vi "setValue.vi"(8 "error in (no error)":errorcluster, 10 "Value":string="000000000000000000000000", 11 "tBSONObjectID in":refnum<class "tBSONObjectID.lvclass">) -> (0 "error out":errorcluster, 3 "tBSONObjectID out":refnum<class "tBSONObjectID.lvclass">)   [LabVIEW 2013, in "BSON.lvlib" / "tBSONObjectID.lvclass"]
uses:
  tBSONObjectID.lvclass
  status.ctl
  tBSONObjectID.lvclass/tBSONObjectID.ctl
  BSON.lvlib
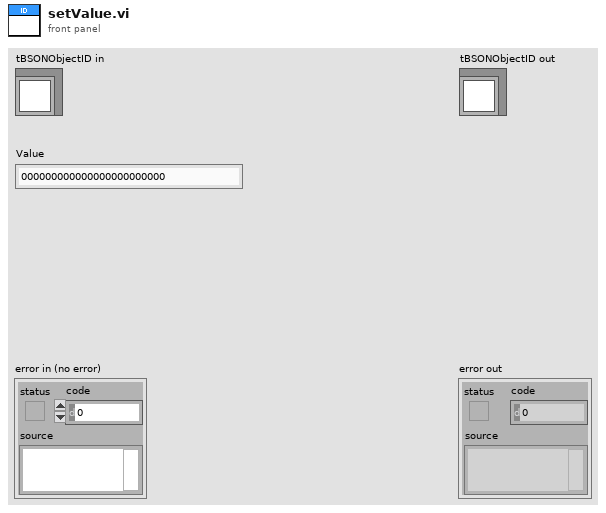
[diagram p1: front panel]
types:
  T1 = typedef "BSON.lvlib/status.ctl" = enum16{"Stream Corrupted or Ended Abruptly", "Incorrect Type In Stream", "ObjectID Invalid", "Method Not Implemented", "Invalid Name", "Invalid URI", "AutoReconnect", "Operation Failed", "Incorrectly Configured", "Cursor Not Found", "Timeout", "Invalid Type", "Empty Name", "Duplicate Name", "MD5Incorrect"}
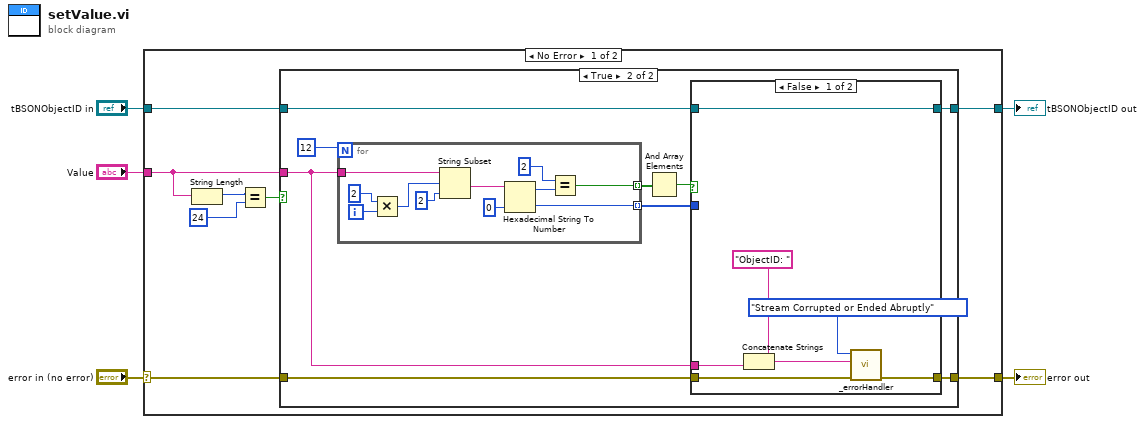
[diagram p0: block diagram]
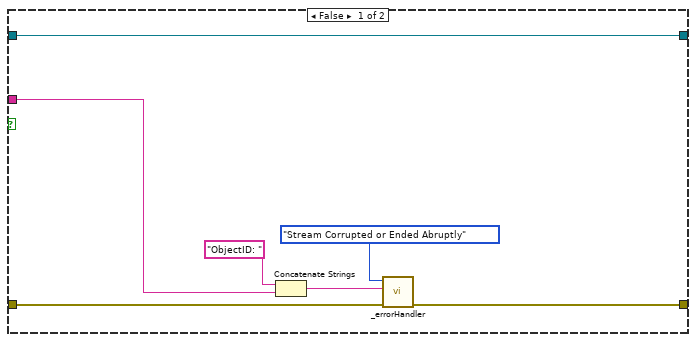
[diagram p2: hidden frame]
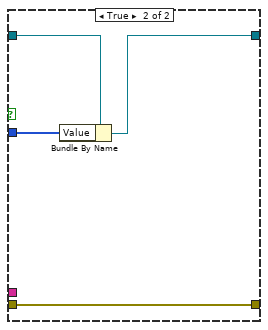
[diagram p3: hidden frame]
diagram:
  n1 = case shown="No Error" "error in (no error)" {
    selector: "error in (no error)" -> [w10 w53]
    tunnel: [w8 w53] -> w4
    tunnel: [w6 w52] -> w2
    tunnel: "tBSONObjectID in" -> [w7 w52]
    tunnel: "Value" -> [w11 _]
    frame No Error {
      n2 = String Length(string=w11) -> (length=w12:i32)
      n3 = Equal?(x=w12, y=24) -> (x = y?=w9:bool)
      n4 = case shown="True" w9 {
        tunnel: w11 -> [w14 w21]
        tunnel: w10 -> [w16 w23]
        tunnel: [w15 w22] -> w8
        tunnel: w7 -> [w20 w28]
        tunnel: [w20 w26] -> w6
        frame False {
          n5 = Concatenate Strings("ObjectID: " ("string"), w14) -> (w17:string)
          n6 = call "_errorHandler.vi"("error in (no error)"=w16, "Additional Text"=w17, "Error Type"=status."Stream Corrupted or Ended Abruptly") -> ("error out"=w15:errorcluster)  [unwired: 8 in]
        }
        frame True {
          n7 = for {
            N: 12 -> [_]
            tunnel: w21 -> [w51]
            tunnel: [w47] -> w27 mode=indexing
            tunnel: [w41] -> w25 mode=indexing
            i -> [w46]
            n8 = Multiply(x=2, y=w46) -> (x*y=w44:i32)
            n9 = String Subset(string=w51, offset (0)=w44, length (rest)=2 ("length (rest)")) -> (substring=w49:string)
            n10 = Hexadecimal String To Number(string=w49, default (0uL)=u8 0 ("default (0 U32)")) -> (offset past number=w43:i32, number=w47:u8)  [unwired: 1 in]
            n11 = Equal?(x=2, y=w43) -> (x = y?=w41:bool)
          }
          n12 = And Array Elements(Boolean array=w25) -> (logical AND=w24:bool)
          n13 = case shown="False" w24 {
            tunnel: w28 -> [w36 w40]
            tunnel: w27 -> [_ w39]
            tunnel: [w36 w38] -> w26
            tunnel: w23 -> [w35 w37]
            tunnel: [w34 w37] -> w22
            tunnel: w21 -> [w32 _]
            frame False {
              n14 = Concatenate Strings("ObjectID: " ("string"), w32) -> (w30:string)
              n15 = call "_errorHandler.vi"("error in (no error)"=w35, "Additional Text"=w30, "Error Type"=status."Stream Corrupted or Ended Abruptly") -> ("error out"=w34:errorcluster)  [unwired: 8 in]
            }
            frame True {
              n16 = Bundle By Name(cluster=w40, "Value"=w39) -> (w38:refnum<class "tBSONObjectID.lvclass">)
            }
          }
        }
      }
    }
    frame Error {
    }
  }
  "error out" <- w4
  "tBSONObjectID out" <- w2
